vi "VISA_I-O.vi"(6 "wait time (ms) [100]":u32=100, 7 "query? [no]":bool, 8 "error in (no error)":errorcluster, 9 "byte count [50]":u32=50, 10 "write buffer":string, 11 "VISA resource name":refnum<visa-resource-name>) -> (0 "error out":errorcluster, 2 "read buffer":string, 3 "VISA resource name out":refnum<visa-resource-name>)   [LabVIEW 2020]
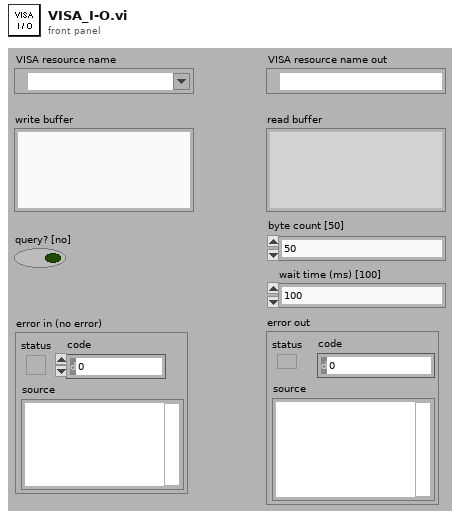
[diagram p1: front panel]
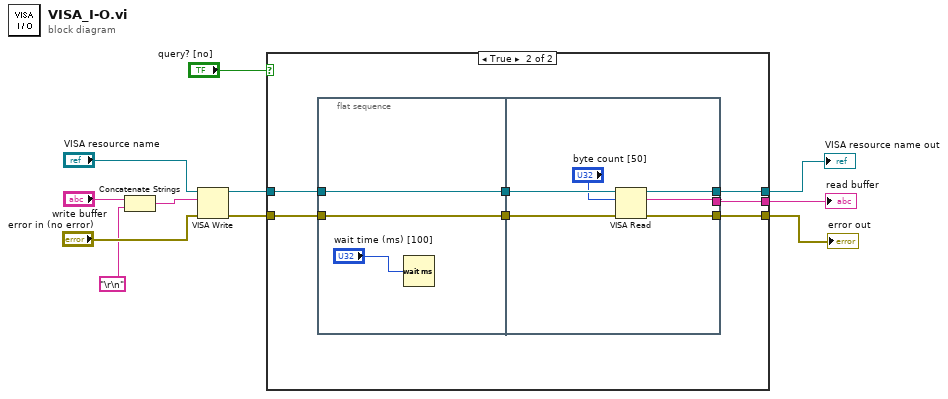
[diagram p0: block diagram]
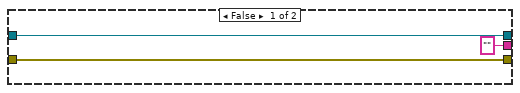
[diagram p2: hidden frame]
diagram:
  n1 = Concatenate Strings("write buffer", "\r\n") -> (w2:string)
  n2 = VISA Write(VISA resource name="VISA resource name", write buffer=w2, error in (no error)="error in (no error)") -> (VISA resource name out=w8:refnum<visa-resource-name>, error out=w7:errorcluster)  [unwired: 1 out]
  n3 = case shown="True" "query? [no]" {
    tunnel: w8 -> [w14 w21]
    tunnel: w7 -> [w13 w20]
    tunnel: [w14 w17] -> w5
    tunnel: [w13 w16] -> w3
    tunnel: ["" ("read buffer") w15] -> w4
    frame False {
    }
    frame True {
      n4 = flat-sequence {
        tunnel: w21 -> [w24]
        tunnel: w20 -> [w23]
        tunnel: [w24] -> w19
        tunnel: [w23] -> w18
        tunnel: w19 -> [w30]
        tunnel: w18 -> [w29]
        tunnel: [w28] -> w17
        tunnel: [w27] -> w16
        tunnel: [w26] -> w15
        frame #0 {
          n5 = Wait (ms)(milliseconds to wait="wait time (ms) [100]") -> ()  [unwired: 1 out]
        }
        frame #1 {
          n6 = VISA Read(VISA resource name=w30, byte count="byte count [50]", error in (no error)=w29) -> (VISA resource name out=w28:refnum<visa-resource-name>, read buffer=w26:string, error out=w27:errorcluster)  [unwired: 1 out]
        }
      }
    }
  }
  "read buffer" <- w4
  "error out" <- w3
  "VISA resource name out" <- w5
